vi "subsystem_getEvent_LoopTimeOutOfRange.vi"(8 "error in (no error)":errorcluster, 11 "ProgrammaticInitialization in":refnum<class "ProgrammaticInitialization.lvclass">) -> (0 "error out":errorcluster, 2 "logevent_LoopTimeOutOfRange":T1, 3 "ProgrammaticInitialization out":refnum<class "ProgrammaticInitialization.lvclass">)   [LabVIEW 2016, in "ProgrammaticInitialization.lvclass"]
uses:
  ProgrammaticInitialization.lvclass
  ts_sallv_sedspectrometer/DataTypes/logevent_loopTimeOutOfRange.ctl
  commandType.ctl
  ProgrammaticInitialization.lvclass/ProgrammaticInitialization.ctl
  ts_sallv_sedspectrometer/DataTypes/logevent_heartbeat.ctl
  ts_sallv_sedspectrometer/SALLV_sedSpectrometer.lvlib
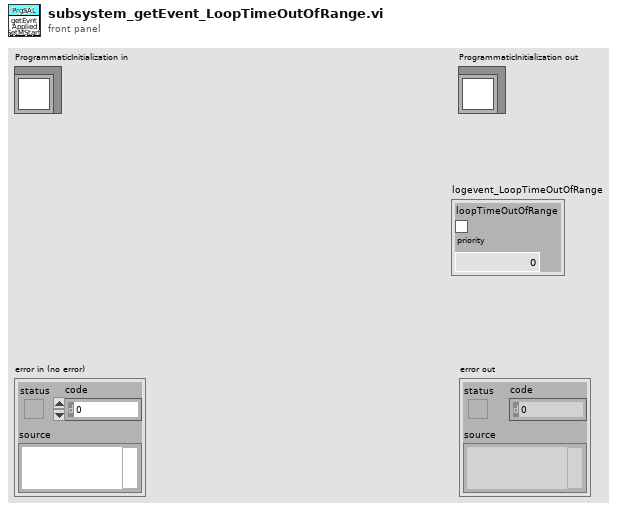
[diagram p1: front panel]
types:
  T1 = typedef "SALLV_sedSpectrometer.lvlib/logevent_loopTimeOutOfRange.ctl" = cluster{"loopTimeOutOfRange":bool, "priority":i32}
  T2 = typedef "ProgrammaticInitialization.lvclass/commandType.ctl" = enum16{"acceptCommand", "ackCommand", "cancelCallback_command", "cancelCallback_logEvent", "cancelCallback", "flushSamplesEvent", "getEvent", "getNextSample", "getResponse", "getSample", "issueCommand", "logEvent", "monitorCommand", "putSample", "registerCallback_command", "registerCallback_logEvent", "registerCallback", "salCommander", "salEvent", "salProcessor", "salTelemetrySub", "waitForCompletion"}
  T3 = typedef "SALLV_sedSpectrometer.lvlib/logevent_heartbeat.ctl" = cluster{"heartbeat":bool, "priority":i32}
  T4 = typedef "SALLV_EXA.lvlib/logevent_Heartbeat.ctl" = cluster{"heartbeat":bool, "priority":i32}
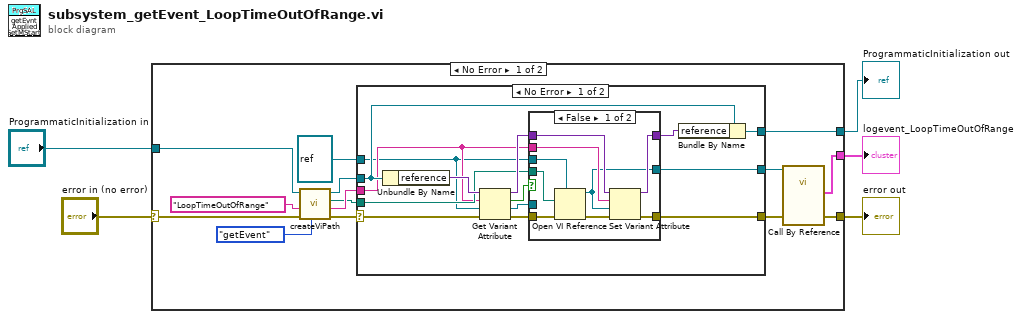
[diagram p0: block diagram]
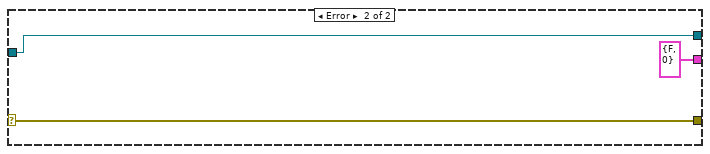
[diagram p4: hidden frame]
diagram:
  n1 = case shown="No Error" "error in (no error)" {
    selector: "error in (no error)" -> [w16 w51]
    tunnel: [w15 w51] -> w4
    tunnel: [w13 w50] -> w2
    tunnel: "ProgrammaticInitialization in" -> [w14 w50]
    tunnel: [w17 T3 {"heartbeat"=FALSE, "priority"=0} ("logevent_Heartbeat_Ctl out")] -> w1
    frame No Error {
      n2 = call "createViPath.vi"("CommandType"=commandType."getEvent", "error in (no error)"=w16, "topic"="LoopTimeOutOfRange", "ProgrammaticInitialization in"=w14) -> ("error out"=w8:errorcluster, "vi name"=w7:string, "path"=w6:path, "ProgrammaticInitialization out"=w9:refnum<class "ProgrammaticInitialization.lvclass">)  [unwired: 4 in]
      n3 = case shown="No Error" w8 {
        selector: w8 -> [w30 w48]
        tunnel: [w29 w48] -> w11
        tunnel: [w25 w47] -> w13
        tunnel: w9 -> [w24 w47]
        tunnel: w7 -> [w22 _]
        tunnel: refnum<vi> refnum ("type specifier VI Refnum (for type only)") -> [w20 w46]
        tunnel: w6 -> [w23 _]
        tunnel: [w21 w46] -> w12
        frame No Error {
          n4 = Unbundle By Name(w24) -> ("reference"=w28:variant)
          n5 = Get Variant Attribute(Variant=w28, name=w22, default value (empty Variant)=w20, error in=w30) -> (duplicate Variant=w27:variant, found=w33:bool, value=w31:refnum<vi>, error out=w32:errorcluster)
          n6 = case shown="False" w33 {
            tunnel: w32 -> [w40 w45]
            tunnel: w31 -> [_ w43]
            tunnel: [w42 w45] -> w29
            tunnel: w27 -> [w35 w44]
            tunnel: [w41 w44] -> w26
            tunnel: w20 -> [w38 _]
            tunnel: w23 -> [w37 _]
            tunnel: w22 -> [w36 _]
            tunnel: [w34 w43] -> w21
            frame False {
              n7 = Open VI Reference(type specifier VI Refnum (for type only)=w38, vi path=w37, error in (no error)=w40) -> (vi reference=w34:refnum<vi>, error out=w39:errorcluster)  [unwired: 3 in]
              n8 = Set Variant Attribute(Variant=w35, name=w36, value=w34, error in=w39) -> (Variant out=w41:variant, error out=w42:errorcluster)  [unwired: 1 out]
            }
            frame True {
            }
          }
          n9 = Bundle By Name(cluster=w24, "reference"=w26) -> (w25:refnum<class "ProgrammaticInitialization.lvclass">)
        }
        frame Error {
        }
      }
      n10 = call-by-ref "?"(reference=w12, "error in (no error)"=w11) -> ("error out"=w15:errorcluster, "logevent_Heartbeat_Ctl out"=w17:T4)  [unwired: 9 in, 3 out]
    }
    frame Error {
    }
  }
  "error out" <- w4
  "ProgrammaticInitialization out" <- w2
  "logevent_LoopTimeOutOfRange" <- w1
